vi "CE GUI Measurement setup.vi"(9 "CE measurement":T1={"Signal frequencies (Hz) T"=[1000.0], "Signal amplitudes (V) T"=[0.707], "Sampling frequencies (Hz) T"=[10000000.0], "Record lengths (multiples of periods) T"=[10000.0], "TWM data root directory"=path "", "TWM mreasurements directories"=[], "Calculate RMS from samples"=FALSE, "Algorithm to use"="TWM-WFFT", "Quantity to read"="rms", "Settle down after AC source change (s) T"=1.0, "Skip PJVS setup"=FALSE, "Measurement template file"=path "", "Row of START keyword T"=0, "Row of STOP keyword T"=0, "Measurement template line T"=[], "Switch position T"=[10000.0], "FR fit mat file T"=path "", "Recalculate-skip already calculated"=FALSE} {"Switch position T" format="%#_3p"; "Record lengths (multiples of periods) T" format="%#_3p"; "Sampling frequencies (Hz) T" format="%#_3p"; "Signal amplitudes (V) T" format="%#_3p"; "Signal frequencies (Hz) T" format="%#_3p"}) -> (3 "CE measurement out":T1={"Signal frequencies (Hz) T"=[1000.0], "Signal amplitudes (V) T"=[0.707], "Sampling frequencies (Hz) T"=[10000000.0], "Record lengths (multiples of periods) T"=[10000.0], "TWM data root directory"=path "", "TWM mreasurements directories"=[], "Calculate RMS from samples"=FALSE, "Algorithm to use"="TWM-WFFT", "Quantity to read"="rms", "Settle down after AC source change (s) T"=1.0, "Skip PJVS setup"=FALSE, "Measurement template file"=path "", "Row of START keyword T"=0, "Row of STOP keyword T"=0, "Measurement template line T"=[], "Switch position T"=[10000.0], "FR fit mat file T"=path "", "Recalculate-skip already calculated"=FALSE} {"Switch position T" format="%#_3p"; "Record lengths (multiples of periods) T" format="%#_3p"; "Sampling frequencies (Hz) T" format="%#_3p"; "Signal amplitudes (V) T" format="%#_3p"; "Signal frequencies (Hz) T" format="%#_3p"})   [LabVIEW 2020]
doc: "deprecated version"
uses:
  CE Measurement/Type definitions/CE measurement.ctl
  <vilib>/Utility/error.llb/Error Cluster From Error Code.vi
  <vilib>/ErrorRing/Error Ring.xnode
  external libraries/varilib/varilib.lvlib
panel:
  in  "Output quantity":string
  in  "Skip PJVS setup":bool caption="Skip setting up PJVS\n(only for standalone\nCE measurement)"
  out "TWM data directories":path[](array[path])
  in  "Save data to folder:":path
  in  "Calculate result":bool=TRUE
  in  "Calculation algorithm":string
  out "Signal amplitudes (V) out":dbl[](array[numeric])
  out "Record lengths (multiples of period)":dbl[](array[numeric])
  out "Sampling frequencies (Hz) out":dbl[](array[numeric])
  out "Signal frequencies (Hz)":dbl[](array[numeric]) caption="List of measurement frequencies" format="%#_7p"
  in  "Settle down after AC\nsource change (s)":dbl=1.0 format="%#_13g"
  out "Measurement points":i32
  in  "Stop freuency (Hz)":i32=7000000 min=1 format="%#_7p"
  in  "Step freuency (Hz)":i32=200000 min=1 format="%#_7p"
  in  "First frequency":i32=1000 format="%#_7p"
  in  "Sampling frequency (Hz)":dbl=10000000.0 format="%#_13p"
  in  "Signal amplitude (V)":dbl=1.0 format="%#_13g"
  in  "Divide frequency by this to\nget number of periods":i32=100
  in  "show connections":bool
  out "gui_elements":refnum<vi>[](array[refnum])
  in  "save_and_quit":bool
  in  "cancel":bool
  # "Who will make\nnice pictures?\n\nwaveforms here"
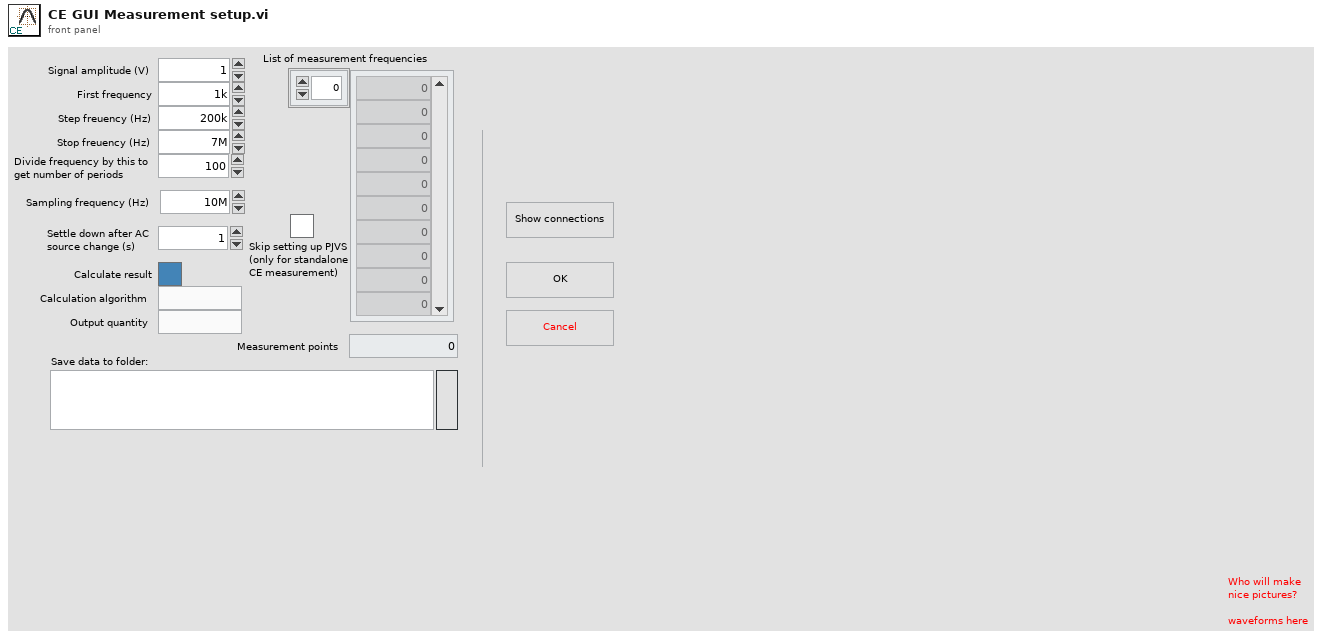
[diagram p1: front panel]
types:
  T1 = typedef "CE measurement.ctl" = cluster{"Signal frequencies (Hz) T":dbl[], "Signal amplitudes (V) T":dbl[], "Sampling frequencies (Hz) T":dbl[], "Record lengths (multiples of periods) T":dbl[], "TWM data root directory":path, "TWM mreasurements directories":path[], "Calculate RMS from samples":bool, "Algorithm to use":string, "Quantity to read":string, "Settle down after AC source change (s) T":dbl, "Skip PJVS setup":bool, "Measurement template file":path, "Row of START keyword T":i32, "Row of STOP keyword T":i32, "Measurement template line T":i32[], "Switch position T":dbl[], "FR fit mat file T":path, "Recalculate-skip already calculated":bool}
  T2 = enum32{"Bad", "Idle", "Run top level", "Running"}
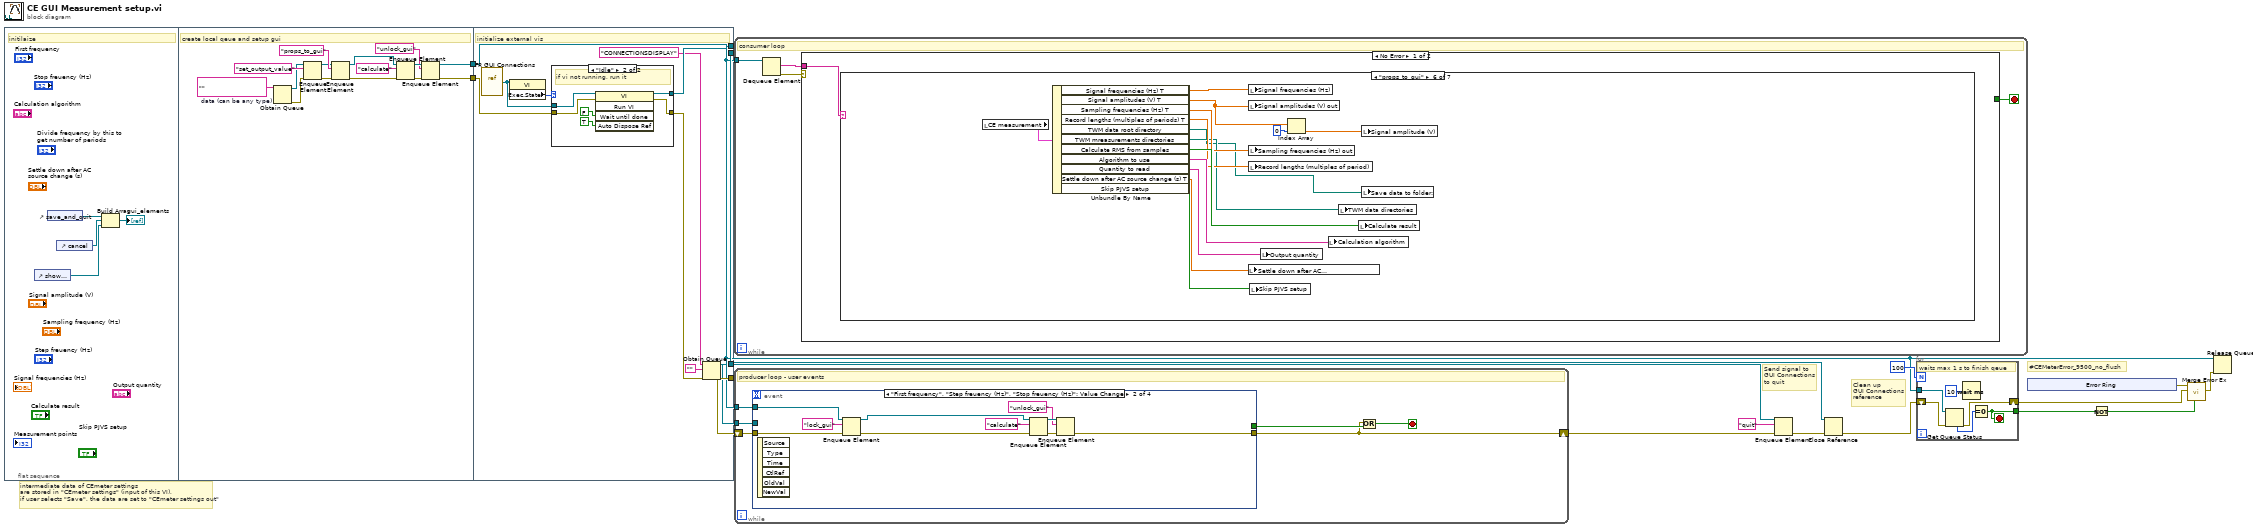
[diagram p0: block diagram]
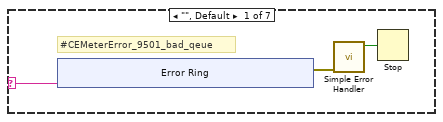
[diagram p3: hidden frame]
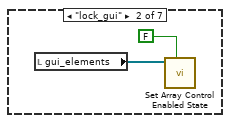
[diagram p4: hidden frame]
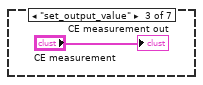
[diagram p5: hidden frame]
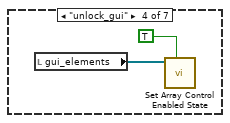
[diagram p6: hidden frame]
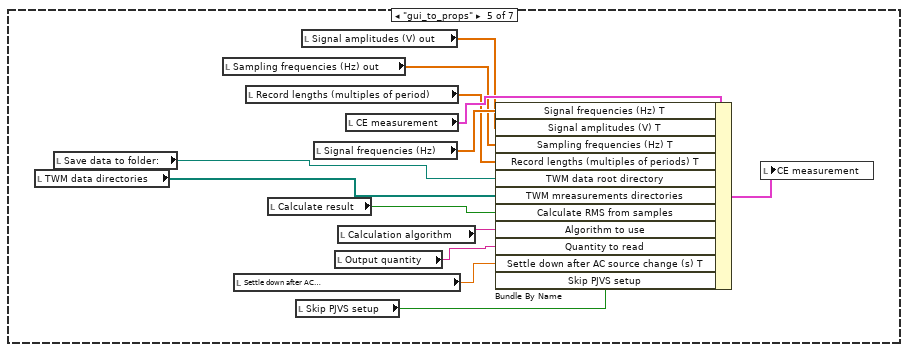
[diagram p7: hidden frame]
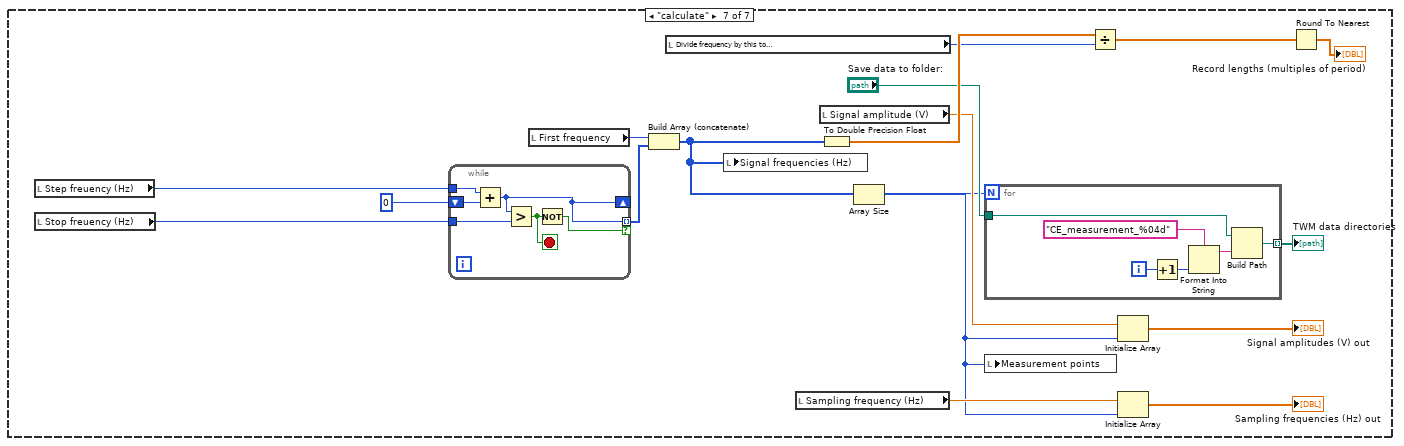
[diagram p8: hidden frame]
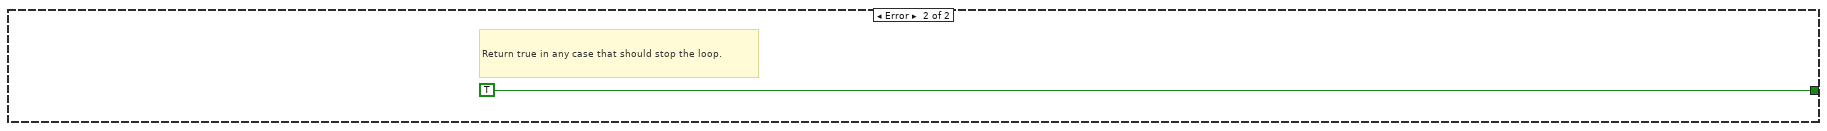
[diagram p9: hidden frame]
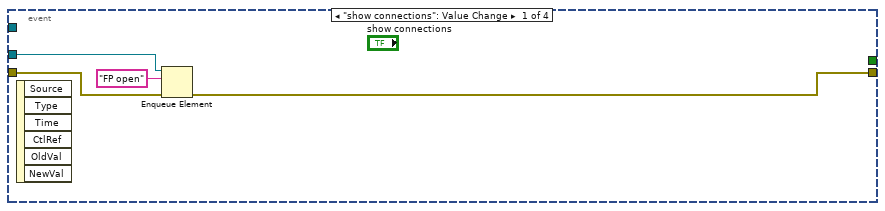
[diagram p10: hidden frame]
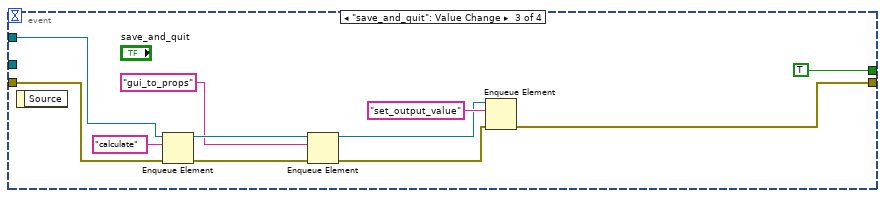
[diagram p11: hidden frame]
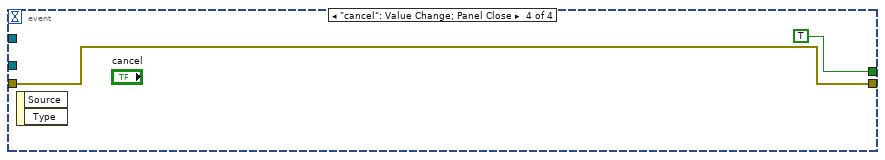
[diagram p12: hidden frame]
diagram:
  # "intermediate data of CEmeter settings\nare stored in \"CEmeter settings\" (input of this VI),\nif user selects \"Save\", the data are set to \"CEmeter settings out\""
  # "Send signal to\nGUI Connections\nto quit"
  # "Clean up\nGUI Connections\nreference"
  # "#CEMeterError_9500_no_flush"
  n1 = flat-sequence {
    tunnel: [w25] -> w9
    tunnel: [w24] -> w1
    tunnel: [w41] -> w10
    tunnel: [w45] -> w4
    tunnel: w9 -> [w44]
    tunnel: [w42] -> w3
    tunnel: [w43] -> w6
    tunnel: w1 -> [w45]
    frame #0 {
      # "initilaize"
      n2 = control-ref of="show connections"() -> (w17:refnum<vi>)
      n3 = control-ref of="save_and_quit"() -> (w20:refnum<vi>)
      n4 = control-ref of="cancel"() -> (w19:refnum<vi>)
      n5 = Build Array(w20, w19, w17) -> (→"gui_elements":refnum<vi>[])
    }
    frame #1 {
      w34 = ""  # data (can be any type)
      # "create local qeue and setup gui"
      n6 = Obtain Queue(element data type=w34) -> (queue out=w27:refnum<queue>, error out=w26:errorcluster)  [unwired: 4 in, 1 out]
      n7 = Enqueue Element(queue=w27, element="set_output_value", error in (no error)=w26) -> (queue out=w29:refnum<queue>, error out=w28:errorcluster)  [unwired: 1 in, 1 out]
      n8 = Enqueue Element(queue=w29, element="props_to_gui", error in (no error)=w28) -> (queue out=w32:refnum<queue>, error out=w33:errorcluster)  [unwired: 1 in, 1 out]
      n9 = Enqueue Element(queue=w32, element="calculate", error in (no error)=w33) -> (queue out=w23:refnum<queue>, error out=w22:errorcluster)  [unwired: 1 in, 1 out]
      n10 = Enqueue Element(queue=w23, element="unlock_gui", error in (no error)=w22) -> (queue out=w24:refnum<queue>, error out=w25:errorcluster)  [unwired: 1 in, 1 out]
    }
    frame #2 {
      # "initialize external vis"
      n11 = vi-ref "FR GUI Connections.vi"() -> (w39:refnum<vi>)
      n12 = property class="VI"(reference=w39) -> ("Exec.State"=w40:T2)  [unwired: 1 in, 2 out]
      n13 = case shown="\"Idle\"" w40 {
        tunnel: [w46 w53] -> w36
        tunnel: w44 -> [w46 w50]
        tunnel: [w47 w49] -> w43
        tunnel: w39 -> [w47 w48]
        frame "Bad", Default {
        }
        frame "Idle" {
          # "if vi not running, run it"
          n14 = invoke class="VI" method="Run VI"(reference=w48, error in=w50, "Wait until done"=FALSE ("Wait Until Done"), "Auto Dispose Ref"=TRUE ("Wait Until Done")) -> (reference out=w49:refnum<vi>, error out=w53:errorcluster)  [unwired: 1 in, 3 out]
        }
      }
      n15 = Obtain Queue(name (unnamed)="CONNECTIONSDISPLAY", element data type="", error in (no error)=w36) -> (queue out=w42:refnum<queue>, error out=w41:errorcluster)  [unwired: 2 in, 1 out]
    }
  }
  n16 = while {
    tunnel: w4 -> [w57]
    stop <- w54 stop-if-true
    # "consumer loop"
    n17 = Dequeue Element(queue=w57) -> (element=w55:string, error out=w56:errorcluster)  [unwired: 2 in, 2 out]
    n18 = case shown="No Error" w56 {
      tunnel: w55 -> [w58 _]
      tunnel: [_ TRUE] -> w54
      frame No Error {
        n19 = case shown="\"props_to_gui\"" w58 {
          selector: w58 -> [w59 _ _ _ _ _ _]
          frame "", Default {
            # "#CEMeterError_9501_bad_qeue"
            n20 = xnode "Error Ring"("parameter 0"=w59) -> ("error out"=w61:errorcluster)
            n21 = call <vilib>:"Simple Error Handler.vi"("error in (no error)"=w61) -> ("error?"=w60:bool)  [unwired: 4 in, 4 out]
            n22 = Stop(stop? (T)=w60) -> ()
          }
          frame "lock_gui" {
            n23 = local read "gui_elements"() -> (w70:refnum<vi>[])
            n24 = call "Set Array Control Enabled State.vi"("enabled (T)"=FALSE, "reference array in"=w70) -> ()  [unwired: 8 in, 2 out]
          }
          frame "set_output_value" {
            "CE measurement out" <- "CE measurement"
          }
          frame "unlock_gui" {
            n25 = local read "gui_elements"() -> (w73:refnum<vi>[])
            n26 = call "Set Array Control Enabled State.vi"("enabled (T)"=TRUE, "reference array in"=w73) -> ()  [unwired: 8 in, 2 out]
          }
          frame "gui_to_props" {
            n27 = local read "TWM data directories"() -> (w79:path[])
            n28 = local read "Save data to folder:"() -> (w76:path)
            n29 = local read "Sampling frequencies (Hz) out"() -> (w82:dbl[])
            n30 = local read "Settle down after AC\nsource change (s)"() -> (w83:dbl)
            n31 = local read "Record lengths (multiples of period)"() -> (w80:dbl[])
            n32 = local read "Calculate result"() -> (w77:bool)
            n33 = local read "Skip PJVS setup"() -> (w75:bool)
            n34 = local read "Signal amplitudes (V) out"() -> (w81:dbl[])
            n35 = local read "Signal frequencies (Hz)"() -> (w84:dbl[])
            n36 = local read "Output quantity"() -> (w74:string)
            n37 = local read "Calculation algorithm"() -> (w78:string)
            n38 = local read "CE measurement"() -> (w85:T1)
            n39 = Bundle By Name(cluster=w85, "Signal frequencies (Hz) T"=w84, "Signal amplitudes (V) T"=w81, "Sampling frequencies (Hz) T"=w82, "Record lengths (multiples of periods) T"=w80, "TWM data root directory"=w76, "TWM mreasurements directories"=w79, "Calculate RMS from samples"=w77, "Algorithm to use"=w78, "Quantity to read"=w74, "Settle down after AC source change (s) T"=w83, "Skip PJVS setup"=w75) -> (w86:T1)
            n40 = local write "CE measurement"(w86) -> ()
          }
          frame "props_to_gui" {
            n41 = local read "CE measurement"() -> (w100:T1)
            n42 = Unbundle By Name(w100) -> ("Signal frequencies (Hz) T"=w94:dbl[], "Signal amplitudes (V) T"=w93:dbl[], "Sampling frequencies (Hz) T"=w95:dbl[], "Record lengths (multiples of periods) T"=w96:dbl[], "TWM data root directory"=w89:path, "TWM mreasurements directories"=w90:path[], "Calculate RMS from samples"=w99:bool, "Algorithm to use"=w98:string, "Quantity to read"=w87:string, "Settle down after AC source change (s) T"=w97:dbl, "Skip PJVS setup"=w88:bool)
            n43 = local write "Settle down after AC\nsource change (s)"(w97) -> ()
            n44 = local write "Signal frequencies (Hz)"(w94) -> ()
            n45 = local write "Signal amplitudes (V) out"(w93) -> ()
            n46 = local write "Sampling frequencies (Hz) out"(w95) -> ()
            n47 = local write "Record lengths (multiples of period)"(w96) -> ()
            n48 = local write "Skip PJVS setup"(w88) -> ()
            n49 = local write "Output quantity"(w87) -> ()
            n50 = Index Array(array=w93, index=0) -> (element=w92:dbl)
            n51 = local write "Calculation algorithm"(w98) -> ()
            n52 = local write "TWM data directories"(w90) -> ()
            n53 = local write "Calculate result"(w99) -> ()
            n54 = local write "Signal amplitude (V)"(w92) -> ()
            n55 = local write "Save data to folder:"(w89) -> ()
          }
          frame "calculate" {
            n56 = local read "Step freuency (Hz)"() -> (w117:i32)
            n57 = local read "Stop freuency (Hz)"() -> (w116:i32)
            n58 = while {
              tunnel: w117 -> [w129]
              tunnel: w116 -> [w128]
              shift-right: [w126] -> _
              shift-left: 0 -> [w127]
              tunnel: [w126] -> w105 mode=indexing if=w125
              stop <- w124 stop-if-true
              n59 = Add(x=w129, y=w127) -> (x+y=w126:i32)
              n60 = Greater?(x=w126, y=w128) -> (0:w124:bool)
              n61 = Not(x=w124) -> (.not. x?=w125:bool)
            }
            n62 = local read "First frequency"() -> (w106:i32)
            n63 = Build Array (concatenate)(w106, w105) -> (w104:i32[])
            n64 = local read "Divide frequency by this to\nget number of periods"() -> (w108:i32)
            n65 = local write "Signal frequencies (Hz)"(w104) -> ()
            n66 = local read "Sampling frequency (Hz)"() -> (w113:dbl)
            n67 = local read "Signal amplitude (V)"() -> (w110:dbl)
            n68 = To Double Precision Float(number=w104) -> (double precision float=w115:dbl[])
            n69 = Array Size(array=w104) -> (size(s)=w101:i32)
            n70 = for {
              N: w101 -> [_]
              tunnel: "Save data to folder:" -> [w120]
              tunnel: [w118] -> w102 mode=indexing
              i -> [w123]
              n71 = Increment(x=w123) -> (x+1=w122:i32)
              n72 = Format Into String(format string="CE_measurement_%04d", w122) -> (resulting string=w119:string)  [unwired: 2 in, 1 out]
              n73 = Build Path(base path=w120, name or relative path=w119) -> (appended path=w118:path)
            }
            "TWM data directories" <- w102
            n74 = local write "Measurement points"(w101) -> ()
            n75 = Divide(x=w115, y=w108) -> (x/y=w114:dbl[])
            n76 = Initialize Array(w110, w101) -> (→"Signal amplitudes (V) out":dbl[])
            n77 = Initialize Array(w113, w101) -> (→"Sampling frequencies (Hz) out":dbl[])
            n78 = Round To Nearest(number=w114) -> (nearest integer value=→"Record lengths (multiples of period)":dbl[])
          }
        }
      }
      frame Error {
        # "Return true in any case that should stop the loop."
      }
    }
  }
  n79 = while {
    shift-right: [w132] -> w5
    shift-left: w10 -> [w135]
    tunnel: w4 -> [w136]
    tunnel: w3 -> [w131]
    stop <- w133 stop-if-true
    # "producer loop - user events"
    n80 = event shown="[1] \"First frequency\", \"Step freuency (Hz)\", \"Stop freuency (Hz)\": Value Change" {
      selector: _ -> [_ _ _ _]
      dyn-events: _ -> [_ _ _ _]
      timeout: _ -> [_ _ _ _]
      tunnel: w136 -> [_ w149 w160 _]
      tunnel: w135 -> [w139 w142 w159 w162]
      tunnel: [w138 w141 w158 w162] -> w132
      tunnel: [_ _ TRUE ("cancel") TRUE ("cancel")] -> w134
      tunnel: w131 -> [w137 _ _ _]
      event "show connections": Value Change {
        n81 = event-data() -> ()  [unwired: 1 in, 6 out]
        n82 = Enqueue Element(queue=w137, element="FP open", error in (no error)=w139) -> (error out=w138:errorcluster)  [unwired: 1 in, 2 out]
      }
      event "First frequency", "Step freuency (Hz)", "Stop freuency (Hz)": Value Change {
        n83 = event-data() -> ()  [unwired: 1 in, 6 out]
        n84 = Enqueue Element(queue=w149, element="lock_gui", error in (no error)=w142) -> (queue out=w148:refnum<queue>, error out=w143:errorcluster)  [unwired: 1 in, 1 out]
        n85 = Enqueue Element(queue=w148, element="calculate", error in (no error)=w143) -> (queue out=w147:refnum<queue>, error out=w144:errorcluster)  [unwired: 1 in, 1 out]
        n86 = Enqueue Element(queue=w147, element="unlock_gui", error in (no error)=w144) -> (error out=w141:errorcluster)  [unwired: 1 in, 2 out]
      }
      event "save_and_quit": Value Change {
        n87 = event-data() -> ()  [unwired: 1 in, 1 out]
        n88 = Enqueue Element(queue=w160, element="calculate", error in (no error)=w159) -> (queue out=w155:refnum<queue>, error out=w156:errorcluster)  [unwired: 1 in, 1 out]
        n89 = Enqueue Element(queue=w155, element="gui_to_props", error in (no error)=w156) -> (queue out=w154:refnum<queue>, error out=w153:errorcluster)  [unwired: 1 in, 1 out]
        n90 = Enqueue Element(queue=w154, element="set_output_value", error in (no error)=w153) -> (error out=w158:errorcluster)  [unwired: 1 in, 2 out]
      }
      event "cancel": Value Change; Panel Close {
        n91 = event-data() -> ()  [unwired: 1 in, 2 out]
      }
    }
    n92 = Or(x=w132, y=w134) -> (x .or. y?=w133:bool)
  }
  n93 = Enqueue Element(queue=w3, element="quit", error in (no error)=w5) -> (error out=w8:errorcluster)  [unwired: 1 in, 2 out]
  n94 = Close Reference(reference=w6, error in (no error)=w8) -> (error out=w2:errorcluster)
  n95 = for {
    N: 100 -> [_]
    tunnel: w4 -> [w169]
    shift-right: [w167] -> w13
    shift-left: w2 -> [w168]
    tunnel: [w164] -> w11
    stop <- w164 stop-if-true
    # "waits max 1 s to finish qeue"
    n96 = Get Queue Status(queue=w169, error in (no error)=w168) -> (error out=w167:errorcluster, # elements in queue=w165:i32)  [unwired: 1 in, 6 out]
    n97 = Wait (ms)(milliseconds to wait=u32 10) -> ()  [unwired: 1 out]
    n98 = Equal To 0?(x=w165) -> (x = 0?=w164:bool)
  }
  n99 = xnode "Error Ring"() -> ("error out"=w14:errorcluster)
  n100 = Not(x=w11) -> (.not. x?=w15:bool)
  n101 = call "Merge Error Ex.vi"("Is error? (False)"=w15, "main error in (no error)"=w13, "second error in"=w14) -> ("error out"=w12:errorcluster)  [unwired: 8 in]
  n102 = Release Queue(queue=w4, error in (no error)=w12) -> ()  [unwired: 1 in, 3 out]
